vi "SetWindowFullscreenMode.vi"(8 "No Error":errorcluster, 9 "Display Mode":T1, 10 "Borderless":bool, 11 "Window [SDL_Window *]":i64) -> (0 "Error Out":errorcluster)   [LabVIEW 2026, in "SDL3.lvlib" / "Video.lvlib"]
doc: "<B>Summary</B>\nSet the display mode to use when a window is visible and fullscreen.\n\n<B>Remarks</B>\nThis only affects the display mode used when the window is fullscreen. To change the window size when the window is not fullscreen, use <B>SDL_SetWindowSize()</B>.\n\nIf the window is currently in the fullscreen state, this request is asynchronous on some windowing systems and the new mode dimensions may not be applied immediately upon the return of this function. If an immediate change is required, call <B>SDL_SyncWindow()</B> to block until the changes have taken effect.\n\nWhen the new mode takes effect, an <B>SDL_EVENT_WINDOW_RESIZED</B> and/or an <B>SDL_EVENT_WINDOW_PIXEL_SIZE_CHANGED</B> event will be emitted with the new mode dimensions."
uses:
  Video.lvlib
  DisplayMode--cluster.ctl
  DisplayID--integer.ctl
  Pixels/PixelFormat--enum.ctl
  7dc3acbc-b491-4a7b-ae7b-9e16c0d03eea.vi
  Pixels/PixelFormatEnumToU32.vi
  7dc3acbc-b491-4a7b-ae7b-9e16c0d03eea.vi/68fb39a4-5dfa-47de-aeef-0ed9366a1549.vi
  <vilib>/Utility/error.llb/Error Cluster From Error Code.vi
  Error/Error.lvlib
  Lib/SDL3.dll
  Pixels/Pixels.lvlib
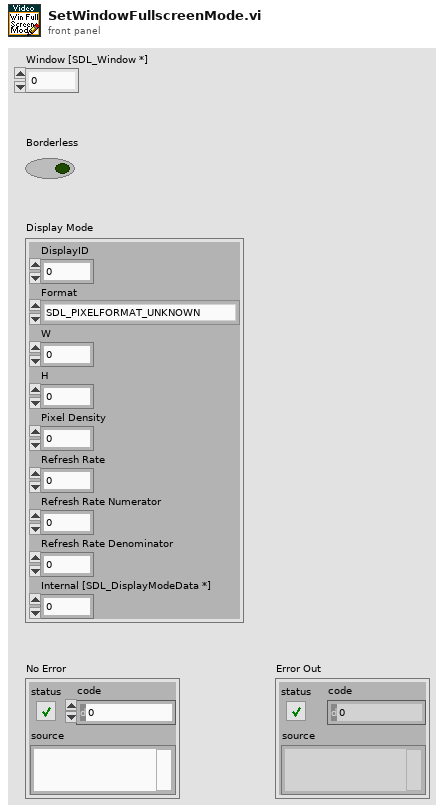
[diagram p1: front panel]
types:
  T1 = typedef "SDL3.lvlib/Video.lvlib/DisplayMode--cluster.ctl" = cluster{"DisplayID":T2, "Format":T3, "W":i32, "H":i32, "Pixel Density":sgl, "Refresh Rate":sgl, "Refresh Rate Numerator":i32, "Refresh Rate Denominator":i32, "Internal [SDL_DisplayModeData *]":i64}
  T2 = typedef "SDL3.lvlib/Video.lvlib/DisplayID--integer.ctl" = u32
  T3 = typedef "SDL3.lvlib/Pixels.lvlib/PixelFormat--enum.ctl" = enum32{"SDL_PIXELFORMAT_UNKNOWN", "SDL_PIXELFORMAT_INDEX1LSB", "SDL_PIXELFORMAT_INDEX1MSB", "SDL_PIXELFORMAT_INDEX2LSB", "SDL_PIXELFORMAT_INDEX2MSB", "SDL_PIXELFORMAT_INDEX4LSB", "SDL_PIXELFORMAT_INDEX4MSB", "SDL_PIXELFORMAT_INDEX8", "SDL_PIXELFORMAT_RGB332", "SDL_PIXELFORMAT_XRGB4444", "SDL_PIXELFORMAT_XBGR4444", "SDL_PIXELFORMAT_XRGB1555", "SDL_PIXELFORMAT_XBGR1555", "SDL_PIXELFORMAT_ARGB4444", "SDL_PIXELFORMAT_RGBA4444", "SDL_PIXELFORMAT_ABGR4444", "SDL_PIXELFORMAT_BGRA4444", "SDL_PIXELFORMAT_ARGB1555", "SDL_PIXELFORMAT_RGBA5551", "SDL_PIXELFORMAT_ABGR1555", "SDL_PIXELFORMAT_BGRA5551", "SDL_PIXELFORMAT_RGB565", "SDL_PIXELFORMAT_BGR565", "SDL_PIXELFORMAT_RGB24", "SDL_PIXELFORMAT_BGR24", "SDL_PIXELFORMAT_XRGB8888", "SDL_PIXELFORMAT_RGBX8888", "SDL_PIXELFORMAT_XBGR8888", "SDL_PIXELFORMAT_BGRX8888", "SDL_PIXELFORMAT_ARGB8888", "SDL_PIXELFORMAT_RGBA8888", "SDL_PIXELFORMAT_ABGR8888", "SDL_PIXELFORMAT_BGRA8888", "SDL_PIXELFORMAT_XRGB2101010", "SDL_PIXELFORMAT_XBGR2101010", "SDL_PIXELFORMAT_ARGB2101010", "SDL_PIXELFORMAT_ABGR2101010", "SDL_PIXELFORMAT_RGB48", "SDL_PIXELFORMAT_BGR48", "SDL_PIXELFORMAT_RGBA64", "SDL_PIXELFORMAT_ARGB64", "SDL_PIXELFORMAT_BGRA64", "SDL_PIXELFORMAT_ABGR64", "SDL_PIXELFORMAT_RGB48_FLOAT", "SDL_PIXELFORMAT_BGR48_FLOAT", "SDL_PIXELFORMAT_RGBA64_FLOAT", "SDL_PIXELFORMAT_ARGB64_FLOAT", "SDL_PIXELFORMAT_BGRA64_FLOAT", "SDL_PIXELFORMAT_ABGR64_FLOAT", "SDL_PIXELFORMAT_RGB96_FLOAT", "SDL_PIXELFORMAT_BGR96_FLOAT", "SDL_PIXELFORMAT_RGBA128_FLOAT", "SDL_PIXELFORMAT_ARGB128_FLOAT", "SDL_PIXELFORMAT_BGRA128_FLOAT", "SDL_PIXELFORMAT_ABGR128_FLOAT", "SDL_PIXELFORMAT_YV12", "SDL_PIXELFORMAT_IYUV", "SDL_PIXELFORMAT_YUY2", "SDL_PIXELFORMAT_UYVY", "SDL_PIXELFORMAT_YVYU", "SDL_PIXELFORMAT_NV12", "SDL_PIXELFORMAT_NV21", "SDL_PIXELFORMAT_P010", "SDL_PIXELFORMAT_EXTERNAL_OES"}
  T4 = typedef "SDL3.lvlib/Video.lvlib/DisplayMode-Internal-Win32--cluster.ctl" = cluster{"DisplayID":T2, "Format":u32, "W":i32, "H":i32, "Pixel Density":sgl, "Refresh Rate":sgl, "Refresh Rate Numerator":i32, "Refresh Rate Denominator":i32, "Internal [SDL_DisplayModeData *]":i32}
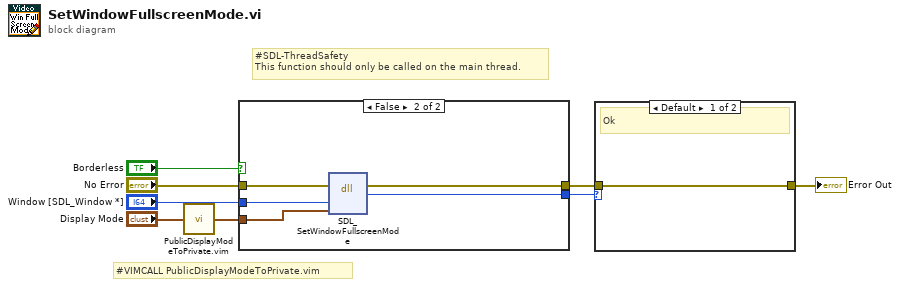
[diagram p0: block diagram]
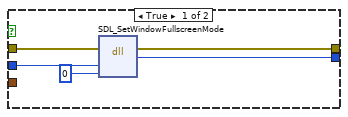
[diagram p2: hidden frame]
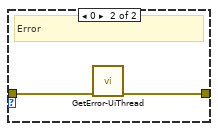
[diagram p3: hidden frame]
diagram:
  # "#VIMCALL PublicDisplayModeToPrivate.vim"
  # "#SDL-ThreadSafety\nThis function should only be called on the main thread."
  n1 = call "PublicDisplayModeToPrivate.vim"("Public Display Mode"="Display Mode") -> ("Private Display Mode"=w3:T4)
  n2 = case shown="False" "Borderless" {
    tunnel: "No Error" -> [w13 w18]
    tunnel: [w12 w17] -> w7
    tunnel: [w11 w16] -> w5
    tunnel: "Window [SDL_Window *]" -> [w10 w15]
    tunnel: w3 -> [_ w14]
    frame True {
      n3 = dll-call lib="C:/Users/saukko/Dev/LV-SDL3/Sources/SDL3/Lib/SDL3.*" fn="SDL_SetWindowFullscreenMode"(error in=w13, "window"=w10, "mode"=i64 0) -> (error out=w12:errorcluster, "return type"=w11:i64)  [unwired: 4 in, 1 out]
    }
    frame False {
      n4 = dll-call lib="C:/Users/saukko/Dev/LV-SDL3/Sources/SDL3/Lib/SDL3.*" fn="SDL_SetWindowFullscreenMode"(error in=w18, "window"=w15, "mode"=w14) -> (error out=w17:errorcluster, "return type"=w16:i64)  [unwired: 4 in, 1 out]
    }
  }
  n5 = case shown="Default" w5 {
    tunnel: w7 -> [w19 w21]
    tunnel: [w19 w20] -> w6
    frame Default {
      # "Ok"
    }
    frame 0 {
      # "Error"
      n6 = call "GetError-UiThread.vi"("No Error"=w21) -> ("error out"=w20:errorcluster)  [unwired: 10 in]
    }
  }
  "Error Out" <- w6
